vi "Core.vi"() -> (19 "Error Out":errorcluster)   [LabVIEW 2017]
uses:
  XDataNode.xnode
panel:
  in  "error in (no error)":errorcluster
  in  "Shutdown":bool
  out "Output Resistance":dbl
  # "Core Module DIagnostics"
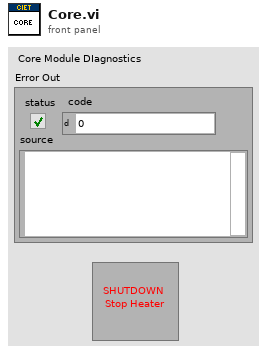
[diagram p1: front panel]
types:
  T1 = cluster{"Expected End [f-1]":u64, "Actual End [f-1]":u64, "Finished Late? [f-1]":bool, "Expected End [i-1]":u64, "Actual End [i-1]":u64, "Finished Late? [i-1]":bool, "Expected Start [i]":u64, "Actual Start [i]":u64, "Expected Start [f]":u64, "Actual Start [f]":u64, "Source Name":string, "Structure Name":string, "Period":i64, "Deadline":i64, "Offset":i64, "Start":i64, "Priority":i32, "Timeout":i32, "Mode":enum32{"No Change", "Process missed periods, maintain original phase", "Discard missed periods, maintain original phase", "Process missed periods, ignore original phase", "Discard missed periods, ignore original phase"}, "Wakeup Reason":enum32{"Normal", "Aborted", "Asynchronous wakeup", "Timing source error", "Timed loop error", "Timeout"}, "Error":errorcluster, "Source Type":string, "Secondary Source Type":string, "Global End Time":u64, "Global Start Time":u64, "Frame Duration":u64, "Iteration Duration":u64, "Assigned CPU":i32, "I/O Scan Engine Mode":u32}
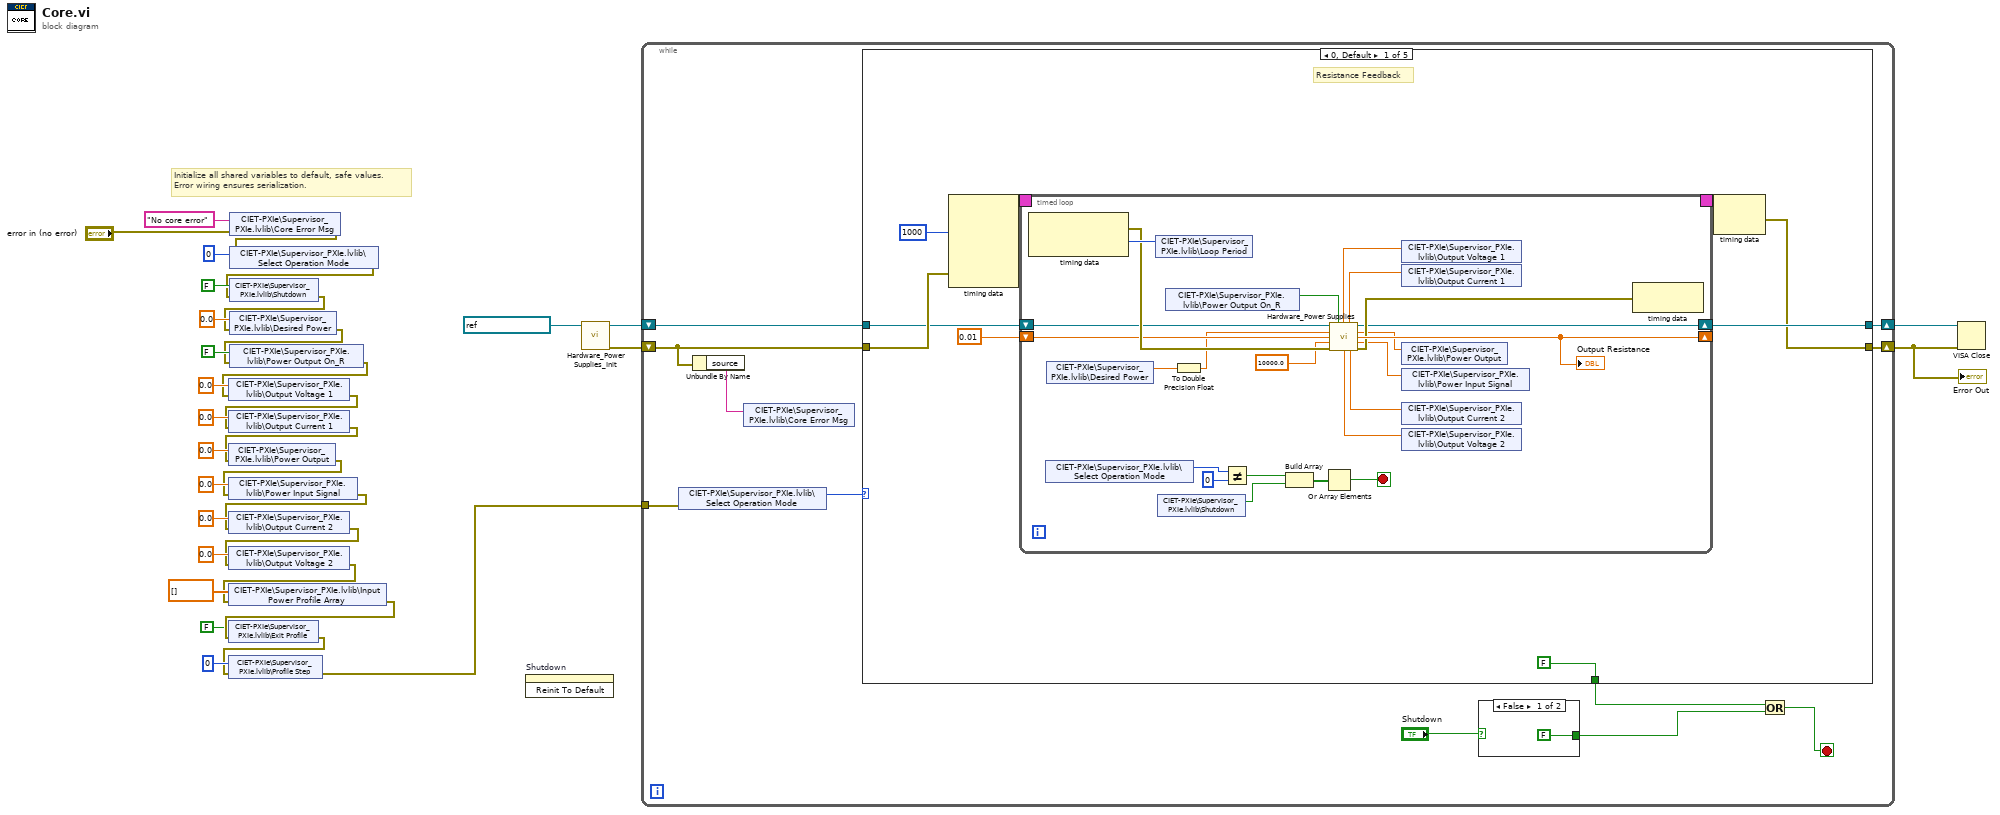
[diagram p0: block diagram]
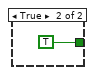
[diagram p2: hidden frame]
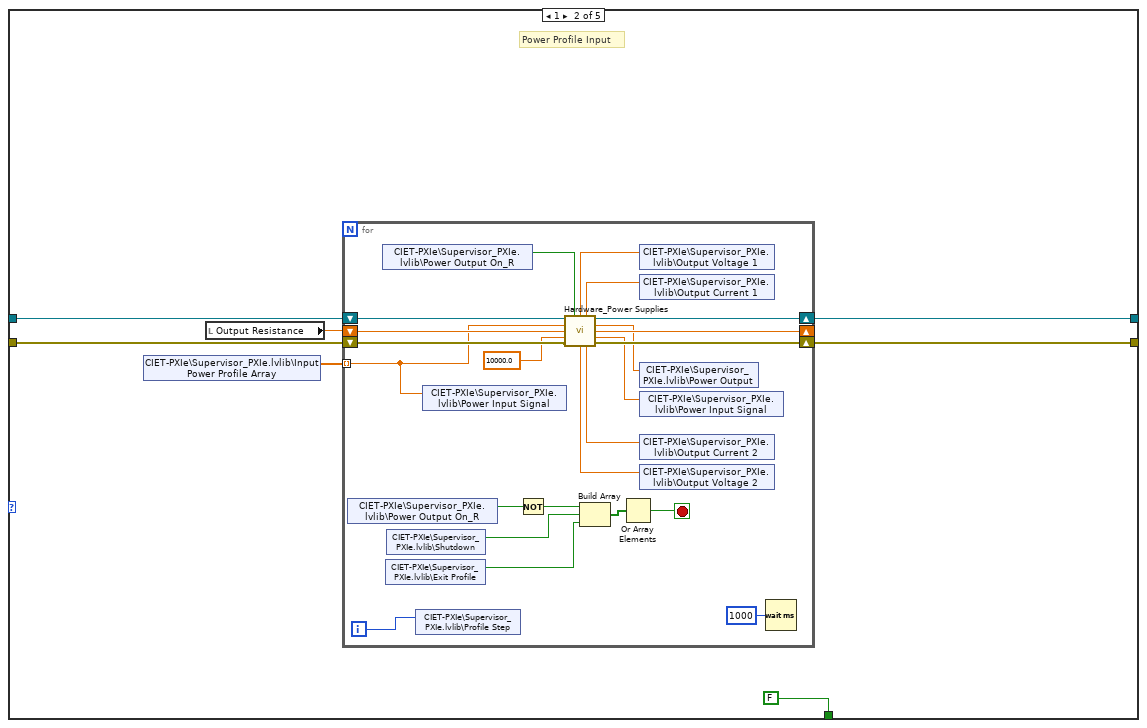
[diagram p3: hidden frame]
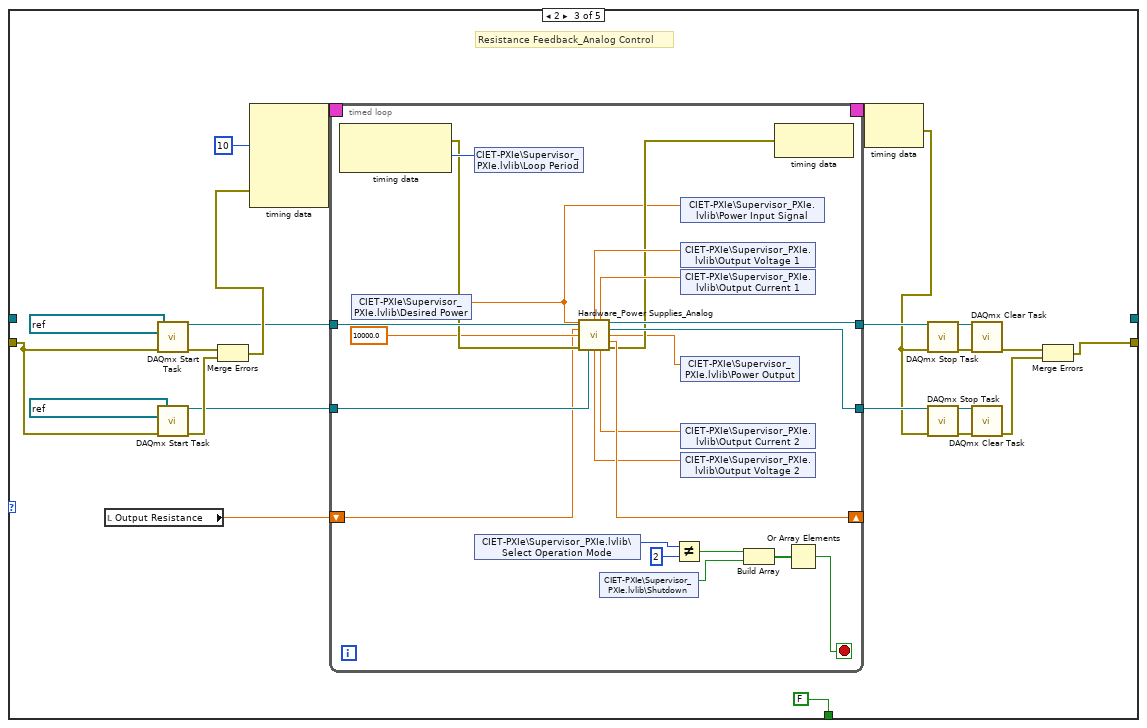
[diagram p4: hidden frame]
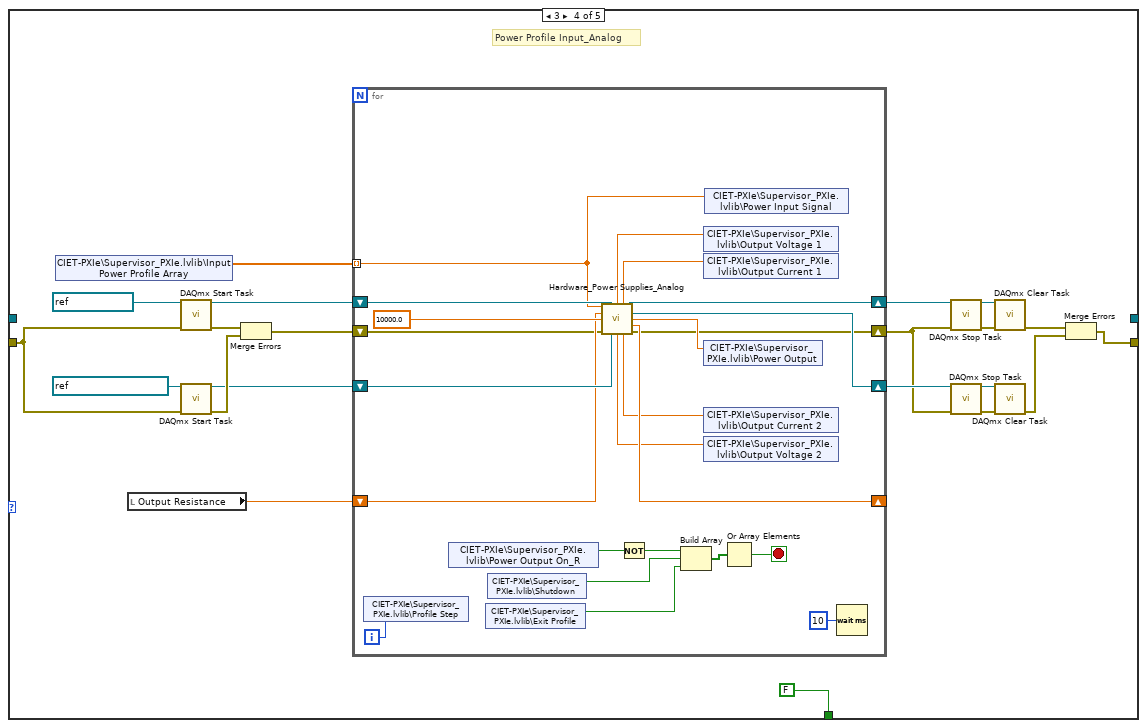
[diagram p5: hidden frame]
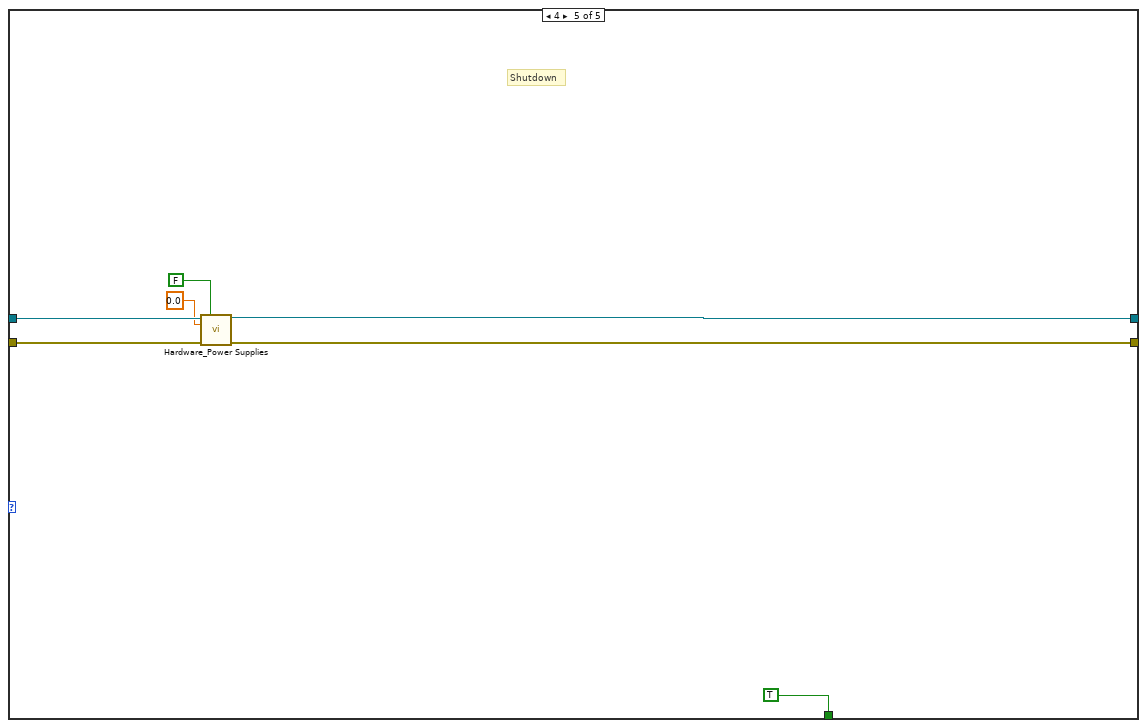
[diagram p6: hidden frame]
diagram:
  # "Initialize all shared variables to default, safe values.\nError wiring ensures serialization."
  n1 = shared-variable "CIET-PXIe\\Supervisor_PXIe.lvlib\\Core Error Msg"("No core error" ("Core Error Msg"), error in="error in (no error)") -> (error out=w25:errorcluster)
  n2 = shared-variable "CIET-PXIe\\Supervisor_PXIe.lvlib\\Select Operation Mode"(u16 0 ("Select Operation Mode"), error in=w25) -> (error out=w24:errorcluster)
  n3 = shared-variable "CIET-PXIe\\Supervisor_PXIe.lvlib\\Shutdown"(FALSE ("Shutdown"), error in=w24) -> (error out=w23:errorcluster)
  n4 = shared-variable "CIET-PXIe\\Supervisor_PXIe.lvlib\\Desired Power"(sgl 0.0 ("Desired Power"), error in=w23) -> (error out=w22:errorcluster)
  n5 = shared-variable "CIET-PXIe\\Supervisor_PXIe.lvlib\\Power Output On_R"(FALSE ("Power Output On_R"), error in=w22) -> (error out=w14:errorcluster)
  n6 = shared-variable "CIET-PXIe\\Supervisor_PXIe.lvlib\\Output Voltage 1"(0.0 ("Output Voltage 1"), error in=w14) -> (error out=w13:errorcluster)
  n7 = shared-variable "CIET-PXIe\\Supervisor_PXIe.lvlib\\Output Current 1"(0.0 ("Output Current 1"), error in=w13) -> (error out=w12:errorcluster)
  n8 = shared-variable "CIET-PXIe\\Supervisor_PXIe.lvlib\\Power Output"(sgl 0.0 ("Power Output"), error in=w12) -> (error out=w11:errorcluster)
  n9 = shared-variable "CIET-PXIe\\Supervisor_PXIe.lvlib\\Power Input Signal"(sgl 0.0 ("Power Input Signal"), error in=w11) -> (error out=w10:errorcluster)
  n10 = shared-variable "CIET-PXIe\\Supervisor_PXIe.lvlib\\Output Current 2"(0.0 ("Output Current 2"), error in=w10) -> (error out=w9:errorcluster)
  n11 = shared-variable "CIET-PXIe\\Supervisor_PXIe.lvlib\\Output Voltage 2"(0.0 ("Output Voltage 2"), error in=w9) -> (error out=w7:errorcluster)
  n12 = shared-variable "CIET-PXIe\\Supervisor_PXIe.lvlib\\Input Power Profile Array"(dbl[] [] ("Input Power Profile Array"), error in=w7) -> (error out=w6:errorcluster)
  n13 = shared-variable "CIET-PXIe\\Supervisor_PXIe.lvlib\\Exit Profile"(FALSE ("Exit Profile"), error in=w6) -> (error out=w3:errorcluster)
  n14 = shared-variable "CIET-PXIe\\Supervisor_PXIe.lvlib\\Profile Step"(0 ("Profile Step"), error in=w3) -> (error out=w1:errorcluster)
  n15 = invoke on="Shutdown" class="Bool (strict)" method="Reinit To Default"() -> ()  [unwired: 3 in, 3 out]
  n16 = call "Hardware_Power Supplies_Init.vi"("VISA name"=refnum<visa-resource-name> "PowerSupply") -> ("Error out"=w2:errorcluster, "VISA out"=w31:refnum<visa-resource-name>)  [unwired: 9 in]
  n17 = while {
    shift-right: [w43] -> w33
    shift-left: w2 -> [w37]
    shift-right: [w44] -> w34
    shift-left: w31 -> [w45]
    tunnel: w1 -> [w35]
    stop <- w39 stop-if-true
    n18 = shared-variable "CIET-PXIe\\Supervisor_PXIe.lvlib\\Select Operation Mode"(error in=w35) -> (w42:u16)  [unwired: 1 out]
    n19 = Unbundle By Name(w37) -> ("source"=w36:string)
    n20 = shared-variable "CIET-PXIe\\Supervisor_PXIe.lvlib\\Core Error Msg"(w36) -> ()  [unwired: 1 in, 1 out]
    n21 = case shown="0, Default" w42 {
      tunnel: w37 -> [w54 w95 w129 w184 w228]
      tunnel: w45 -> [w53 w98 _ _ w227]
      tunnel: [w51 w97 _ _ w226] -> w44
      tunnel: [w50 w94 w134 w183 w225] -> w43
      tunnel: [FALSE ("Shutdown") FALSE ("Shutdown") FALSE ("Shutdown") FALSE ("Shutdown") TRUE ("Shutdown")] -> w41
      frame 0, Default {
        # "Resistance Feedback"
        n22 = node-c288(i64 1000 ("Period"), w54) -> (w56:T1)  [unwired: 3 in]
        n23 = timed-loop {
          timing: w56 -> [_]
          timing-out: [_] -> w55
          shift-right: [w64] -> w51
          shift-left: w53 -> [w71]
          shift-right: [w68] -> _
          shift-left: 0.01 -> [w70]
          stop <- w76 stop-if-true
          n24 = node-c288() -> (w72:errorcluster, w75:i64)  [unwired: 1 in]
          n25 = shared-variable "CIET-PXIe\\Supervisor_PXIe.lvlib\\Select Operation Mode"() -> (w74:u16)  [unwired: 1 in, 1 out]
          n26 = shared-variable "CIET-PXIe\\Supervisor_PXIe.lvlib\\Desired Power"() -> (w58:sgl)  [unwired: 1 in, 1 out]
          n27 = shared-variable "CIET-PXIe\\Supervisor_PXIe.lvlib\\Loop Period"(w75) -> ()  [unwired: 1 in, 1 out]
          n28 = shared-variable "CIET-PXIe\\Supervisor_PXIe.lvlib\\Shutdown"() -> (w73:bool)  [unwired: 1 in, 1 out]
          n29 = shared-variable "CIET-PXIe\\Supervisor_PXIe.lvlib\\Power Output On_R"() -> (w63:bool)  [unwired: 1 in, 1 out]
          n30 = To Double Precision Float(number=w58) -> (double precision float=w57:dbl)
          n31 = Not Equal?(x=w74, y=u16 0) -> (x != y?=w78:bool)
          n32 = Build Array(w78, w73) -> (w77:bool[])
          n33 = Or Array Elements(Boolean array=w77) -> (logical OR=w76:bool)
          n34 = call "Hardware_Power Supplies.vi"("Input VISA"=w71, "Power Output ON"=w63, "Desired Power"=w57, "Input Resistance"=w70, "Maximum Power Limit"=10000.0, "Input Error"=w72) -> ("Output Voltage 1"=w62:dbl, "Output Current 1"=w61:dbl, "Output VISA"=w64:refnum<visa-resource-name>, "Output Power"=w65:dbl, "Output Resistance"=w68:dbl, "Input Power"=w66:dbl, "Output Voltage 2"=w59:dbl, "Output Current 2"=w60:dbl, "Output Error"=w67:errorcluster)  [unwired: 1 in]
          "Output Resistance" <- w68
          n35 = shared-variable "CIET-PXIe\\Supervisor_PXIe.lvlib\\Output Voltage 1"(w62) -> ()  [unwired: 1 in, 1 out]
          n36 = shared-variable "CIET-PXIe\\Supervisor_PXIe.lvlib\\Output Current 1"(w61) -> ()  [unwired: 1 in, 1 out]
          n37 = shared-variable "CIET-PXIe\\Supervisor_PXIe.lvlib\\Power Output"(w65) -> ()  [unwired: 1 in, 1 out]
          n38 = shared-variable "CIET-PXIe\\Supervisor_PXIe.lvlib\\Power Input Signal"(w66) -> ()  [unwired: 1 in, 1 out]
          n39 = shared-variable "CIET-PXIe\\Supervisor_PXIe.lvlib\\Output Current 2"(w60) -> ()  [unwired: 1 in, 1 out]
          n40 = shared-variable "CIET-PXIe\\Supervisor_PXIe.lvlib\\Output Voltage 2"(w59) -> ()  [unwired: 1 in, 1 out]
          n41 = node-c288(w67) -> ()  [unwired: 1 out]
        }
        n42 = node-c288(w55) -> (w50:errorcluster)
      }
      frame 1 {
        # "Power Profile Input"
        n43 = shared-variable "CIET-PXIe\\Supervisor_PXIe.lvlib\\Input Power Profile Array"() -> (w92:dbl[])  [unwired: 1 in, 1 out]
        n44 = local read "Output Resistance"() -> (w96:dbl)
        n45 = for {
          shift-right: [w113] -> w97
          shift-left: w98 -> [w114]
          shift-right: [w112] -> w94
          shift-left: w95 -> [w111]
          tunnel: w92 -> [w99] mode=indexing
          shift-right: [w105] -> _
          shift-left: w96 -> [w104]
          i -> [w115]
          stop <- w119 stop-if-true
          n46 = shared-variable "CIET-PXIe\\Supervisor_PXIe.lvlib\\Power Output On_R"() -> (w117:bool)  [unwired: 1 in, 1 out]
          n47 = shared-variable "CIET-PXIe\\Supervisor_PXIe.lvlib\\Power Output On_R"() -> (w110:bool)  [unwired: 1 in, 1 out]
          n48 = shared-variable "CIET-PXIe\\Supervisor_PXIe.lvlib\\Exit Profile"() -> (w100:bool)  [unwired: 1 in, 1 out]
          n49 = shared-variable "CIET-PXIe\\Supervisor_PXIe.lvlib\\Shutdown"() -> (w116:bool)  [unwired: 1 in, 1 out]
          n50 = shared-variable "CIET-PXIe\\Supervisor_PXIe.lvlib\\Profile Step"(w115) -> ()  [unwired: 1 in, 1 out]
          n51 = shared-variable "CIET-PXIe\\Supervisor_PXIe.lvlib\\Power Input Signal"(w99) -> ()  [unwired: 1 in, 1 out]
          n52 = Not(x=w117) -> (.not. x?=w118:bool)
          n53 = call "Hardware_Power Supplies.vi"("Input VISA"=w114, "Power Output ON"=w110, "Desired Power"=w99, "Input Resistance"=w104, "Maximum Power Limit"=10000.0, "Input Error"=w111) -> ("Output Voltage 1"=w109:dbl, "Output Current 1"=w108:dbl, "Output VISA"=w113:refnum<visa-resource-name>, "Output Power"=w102:dbl, "Output Resistance"=w105:dbl, "Input Power"=w101:dbl, "Output Voltage 2"=w107:dbl, "Output Current 2"=w106:dbl, "Output Error"=w112:errorcluster)  [unwired: 1 in]
          n54 = Build Array(w118, w116, w100) -> (w121:bool[])
          n55 = Or Array Elements(Boolean array=w121) -> (logical OR=w119:bool)
          n56 = shared-variable "CIET-PXIe\\Supervisor_PXIe.lvlib\\Output Voltage 1"(w109) -> ()  [unwired: 1 in, 1 out]
          n57 = shared-variable "CIET-PXIe\\Supervisor_PXIe.lvlib\\Output Current 1"(w108) -> ()  [unwired: 1 in, 1 out]
          n58 = shared-variable "CIET-PXIe\\Supervisor_PXIe.lvlib\\Power Output"(w102) -> ()  [unwired: 1 in, 1 out]
          n59 = shared-variable "CIET-PXIe\\Supervisor_PXIe.lvlib\\Power Input Signal"(w101) -> ()  [unwired: 1 in, 1 out]
          n60 = shared-variable "CIET-PXIe\\Supervisor_PXIe.lvlib\\Output Current 2"(w106) -> ()  [unwired: 1 in, 1 out]
          n61 = shared-variable "CIET-PXIe\\Supervisor_PXIe.lvlib\\Output Voltage 2"(w107) -> ()  [unwired: 1 in, 1 out]
          n62 = Wait (ms)(milliseconds to wait=u32 1000) -> ()  [unwired: 1 out]
        }
      }
      frame 2 {
        # "Resistance Feedback_Analog Control"
        n63 = local read "Output Resistance"() -> (w126:dbl)
        n64 = call "DAQmx Start Task.vi"("task/channels in"=refnum<k21> "CIET-Power-Control", "error in"=w129) -> ("task out"=w128:refnum<k21>, "error out"=w144:errorcluster)  [unwired: 12 in]
        n65 = call "DAQmx Start Task.vi"("task/channels in"=refnum<k21> "CIET-Power-Monitor", "error in"=w129) -> ("task out"=w127:refnum<k21>, "error out"=w143:errorcluster)  [unwired: 12 in]
        n66 = Merge Errors(w144, w143) -> (w130:errorcluster)
        n67 = node-c288(i64 10 ("Period"), w130) -> (w133:T1)  [unwired: 3 in]
        n68 = timed-loop {
          timing: w133 -> [_]
          timing-out: [_] -> w132
          shift-right: [w160] -> _
          shift-left: w126 -> [w161]
          tunnel: w128 -> [w165]
          tunnel: [w159] -> w125
          tunnel: w127 -> [w164]
          tunnel: [w158] -> w124
          stop <- w146 stop-if-true
          n69 = node-c288() -> (w163:errorcluster, w166:i64)  [unwired: 1 in]
          n70 = shared-variable "CIET-PXIe\\Supervisor_PXIe.lvlib\\Desired Power"() -> (w145:sgl)  [unwired: 1 in, 1 out]
          n71 = shared-variable "CIET-PXIe\\Supervisor_PXIe.lvlib\\Loop Period"(w166) -> ()  [unwired: 1 in, 1 out]
          n72 = shared-variable "CIET-PXIe\\Supervisor_PXIe.lvlib\\Select Operation Mode"() -> (w148:u16)  [unwired: 1 in, 1 out]
          n73 = call "Hardware_Power Supplies_Analog.vi"("Desired Power"=w145, "Task In_1"=w165, "Input Resistance"=w161, "Maximum Power Limit"=10000.0, "Error In"=w163, "Task In_2"=w164) -> ("Output Voltage 1"=w157:dbl, "Output Current 1"=w156:dbl, "Task Out_1"=w159:refnum<k21>, "Task Out_2"=w158:refnum<k21>, "Output Power"=w152:dbl, "Output Resistance"=w160:dbl, "Output Voltage 2"=w155:dbl, "Output Current 2"=w154:dbl, "Error Out"=w153:errorcluster)  [unwired: 1 in]
          n74 = shared-variable "CIET-PXIe\\Supervisor_PXIe.lvlib\\Shutdown"() -> (w147:bool)  [unwired: 1 in, 1 out]
          n75 = Not Equal?(x=w148, y=u16 2) -> (x != y?=w150:bool)
          n76 = shared-variable "CIET-PXIe\\Supervisor_PXIe.lvlib\\Power Input Signal"(w145) -> ()  [unwired: 1 in, 1 out]
          n77 = shared-variable "CIET-PXIe\\Supervisor_PXIe.lvlib\\Output Voltage 1"(w157) -> ()  [unwired: 1 in, 1 out]
          n78 = shared-variable "CIET-PXIe\\Supervisor_PXIe.lvlib\\Output Current 1"(w156) -> ()  [unwired: 1 in, 1 out]
          n79 = shared-variable "CIET-PXIe\\Supervisor_PXIe.lvlib\\Power Output"(w152) -> ()  [unwired: 1 in, 1 out]
          n80 = shared-variable "CIET-PXIe\\Supervisor_PXIe.lvlib\\Output Current 2"(w154) -> ()  [unwired: 1 in, 1 out]
          n81 = shared-variable "CIET-PXIe\\Supervisor_PXIe.lvlib\\Output Voltage 2"(w155) -> ()  [unwired: 1 in, 1 out]
          n82 = Build Array(w150, w147) -> (w149:bool[])
          n83 = node-c288(w153) -> ()  [unwired: 1 out]
          n84 = Or Array Elements(Boolean array=w149) -> (logical OR=w146:bool)
        }
        n85 = node-c288(w132) -> (w122:errorcluster)
        n86 = call "DAQmx Stop Task.vi"("task/channels in"=w125, "error in"=w122) -> ("task out"=w140:refnum<k21>, "error out"=w139:errorcluster)  [unwired: 12 in]
        n87 = call "DAQmx Stop Task.vi"("task/channels in"=w124, "error in"=w122) -> ("task out"=w138:refnum<k21>, "error out"=w137:errorcluster)  [unwired: 12 in]
        n88 = call "DAQmx Clear Task.vi"("task in"=w140, "error in"=w139) -> ("error out"=w136:errorcluster)  [unwired: 13 in]
        n89 = call "DAQmx Clear Task.vi"("task in"=w138, "error in"=w137) -> ("error out"=w135:errorcluster)  [unwired: 13 in]
        n90 = Merge Errors(w136, w135) -> (w134:errorcluster)
      }
      frame 3 {
        # "Power Profile Input_Analog"
        n91 = shared-variable "CIET-PXIe\\Supervisor_PXIe.lvlib\\Input Power Profile Array"() -> (w180:dbl[])  [unwired: 1 in, 1 out]
        n92 = local read "Output Resistance"() -> (w187:dbl)
        n93 = call "DAQmx Start Task.vi"("task/channels in"=refnum<k21> "PowerOut", "error in"=w184) -> ("task out"=w189:refnum<k21>, "error out"=w199:errorcluster)  [unwired: 12 in]
        n94 = call "DAQmx Start Task.vi"("task/channels in"=refnum<k21> "PowerMonitor_V", "error in"=w184) -> ("task out"=w188:refnum<k21>, "error out"=w198:errorcluster)  [unwired: 12 in]
        n95 = Merge Errors(w199, w198) -> (w182:errorcluster)
        n96 = for {
          shift-right: [w218] -> _
          shift-left: w187 -> [w219]
          shift-right: [w217] -> w186
          shift-left: w189 -> [w222]
          shift-right: [w216] -> w185
          shift-left: w188 -> [w221]
          shift-right: [w209] -> w181
          shift-left: w182 -> [w210]
          tunnel: w180 -> [w200] mode=indexing
          i -> [w204]
          stop <- w203 stop-if-true
          n97 = shared-variable "CIET-PXIe\\Supervisor_PXIe.lvlib\\Profile Step"(w204) -> ()  [unwired: 1 in, 1 out]
          n98 = shared-variable "CIET-PXIe\\Supervisor_PXIe.lvlib\\Power Output On_R"() -> (w206:bool)  [unwired: 1 in, 1 out]
          n99 = shared-variable "CIET-PXIe\\Supervisor_PXIe.lvlib\\Exit Profile"() -> (w201:bool)  [unwired: 1 in, 1 out]
          n100 = shared-variable "CIET-PXIe\\Supervisor_PXIe.lvlib\\Shutdown"() -> (w205:bool)  [unwired: 1 in, 1 out]
          n101 = call "Hardware_Power Supplies_Analog.vi"("Desired Power"=w200, "Task In_1"=w222, "Input Resistance"=w219, "Maximum Power Limit"=10000.0, "Error In"=w210, "Task In_2"=w221) -> ("Output Voltage 1"=w215:dbl, "Output Current 1"=w214:dbl, "Task Out_1"=w217:refnum<k21>, "Task Out_2"=w216:refnum<k21>, "Output Power"=w211:dbl, "Output Resistance"=w218:dbl, "Output Voltage 2"=w213:dbl, "Output Current 2"=w212:dbl, "Error Out"=w209:errorcluster)  [unwired: 1 in]
          n102 = Not(x=w206) -> (.not. x?=w207:bool)
          n103 = Build Array(w207, w205, w201) -> (w208:bool[])
          n104 = shared-variable "CIET-PXIe\\Supervisor_PXIe.lvlib\\Output Voltage 1"(w215) -> ()  [unwired: 1 in, 1 out]
          n105 = shared-variable "CIET-PXIe\\Supervisor_PXIe.lvlib\\Output Current 1"(w214) -> ()  [unwired: 1 in, 1 out]
          n106 = shared-variable "CIET-PXIe\\Supervisor_PXIe.lvlib\\Power Output"(w211) -> ()  [unwired: 1 in, 1 out]
          n107 = shared-variable "CIET-PXIe\\Supervisor_PXIe.lvlib\\Output Current 2"(w212) -> ()  [unwired: 1 in, 1 out]
          n108 = shared-variable "CIET-PXIe\\Supervisor_PXIe.lvlib\\Output Voltage 2"(w213) -> ()  [unwired: 1 in, 1 out]
          n109 = shared-variable "CIET-PXIe\\Supervisor_PXIe.lvlib\\Power Input Signal"(w200) -> ()  [unwired: 1 in, 1 out]
          n110 = Or Array Elements(Boolean array=w208) -> (logical OR=w203:bool)
          n111 = Wait (ms)(milliseconds to wait=u32 10) -> ()  [unwired: 1 out]
        }
        n112 = call "DAQmx Stop Task.vi"("task/channels in"=w186, "error in"=w181) -> ("task out"=w195:refnum<k21>, "error out"=w194:errorcluster)  [unwired: 12 in]
        n113 = call "DAQmx Stop Task.vi"("task/channels in"=w185, "error in"=w181) -> ("task out"=w193:refnum<k21>, "error out"=w192:errorcluster)  [unwired: 12 in]
        n114 = call "DAQmx Clear Task.vi"("task in"=w195, "error in"=w194) -> ("error out"=w191:errorcluster)  [unwired: 13 in]
        n115 = call "DAQmx Clear Task.vi"("task in"=w193, "error in"=w192) -> ("error out"=w190:errorcluster)  [unwired: 13 in]
        n116 = Merge Errors(w191, w190) -> (w183:errorcluster)
      }
      frame 4 {
        # "Shutdown"
        n117 = call "Hardware_Power Supplies.vi"("Input VISA"=w227, "Power Output ON"=FALSE, "Desired Power"=0.0, "Input Error"=w228) -> ("Output VISA"=w226:refnum<visa-resource-name>, "Output Error"=w225:errorcluster)  [unwired: 3 in, 7 out]
      }
    }
    n118 = case shown="False" "Shutdown" {
      tunnel: [FALSE ("Shutdown") TRUE ("Shutdown")] -> w40
      frame False {
      }
      frame True {
      }
    }
    n119 = Or(x=w41, y=w40) -> (x .or. y?=w39:bool)
  }
  "Error Out" <- w33
  n120 = VISA Close(VISA resource name=w34, error in (no error)=w33) -> ()  [unwired: 1 out]
